vi "Read Bid.vi"(8 "error in (no error)":errorcluster, 11 "CardHand in":refnum<class "CardHand.lvclass">) -> (0 "error out":errorcluster, 2 "Bid":i32, 3 "CardHand out":refnum<class "CardHand.lvclass">)   [LabVIEW 2021, in "2023.lvlib" / "CardHand.lvclass"]
uses:
  CardHand.lvclass
  CardHand.lvclass/CardHand.ctl
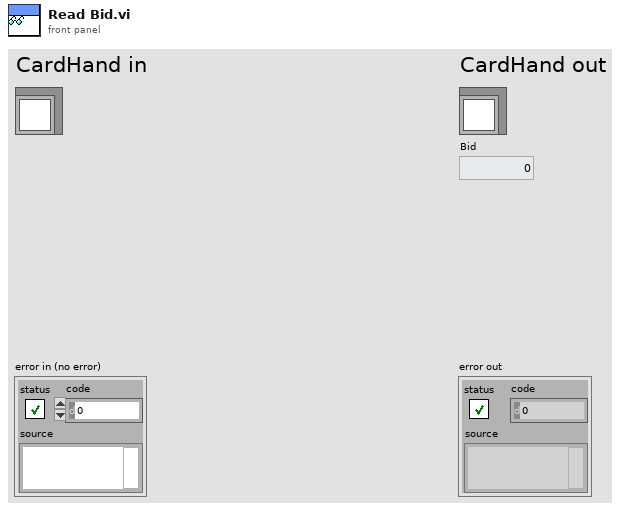
[diagram p1: front panel]
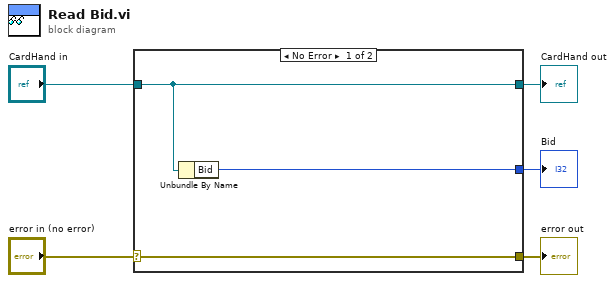
[diagram p0: block diagram]
diagram:
  n1 = case shown="No Error" "error in (no error)" {
    selector: "error in (no error)" -> [w8 w9]
    tunnel: [w8 w9] -> w4
    tunnel: [w7 w10] -> w2
    tunnel: "CardHand in" -> [w7 w10]
    tunnel: [w6 _] -> w1
    frame No Error {
      n2 = Unbundle By Name(w7) -> ("Bid"=w6:i32)
    }
    frame Error {
    }
  }
  "error out" <- w4
  "CardHand out" <- w2
  "Bid" <- w1
